vi "LJUD UE9RAW SingleIO.vi"(5 "Comm Settings":T1={"Open LabJack "=TRUE, "Use USB"=TRUE, "IP Address"="192.168.1.209", "PortA"=52360, "PortB"=0}, 8 "error in (no error)":errorcluster, 10 "Write Parameters":T3 {"IOType" items=["Digital Bit In", "Digital Bit Out", "Digital Port In", "Digital Port Out", "Analog In", "Analog Out"]}, 11 "Handle In":i32) -> (0 "error out":errorcluster, 2 "Read Parameters":T2 {"IOType" items=["Digital Bit In", "Digital Bit Out", "Digital Port In", "Digital Port Out", "Analog In", "Analog Out"]}, 3 "Handle Out":i32)   [LabVIEW 2021]
panel:
  # "Digital Port\nChannel:\n0  =  FIO\n1  =  EIO\n2  =  CIO\n3  =  MIO"
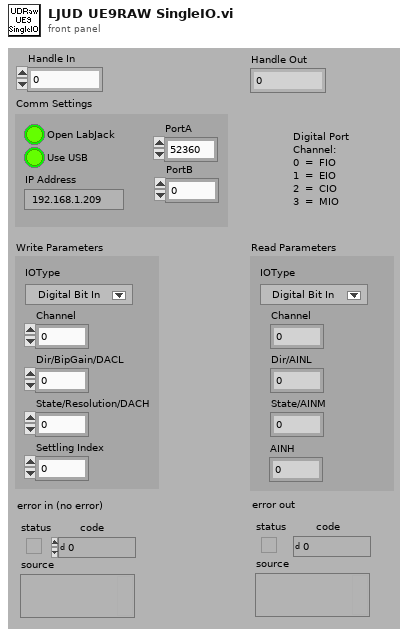
[diagram p1: front panel]
types:
  T1 = cluster{"Open LabJack ":bool, "Use USB":bool, "IP Address":string, "PortA":u16, "PortB":u16}
  T2 = cluster{"IOType":u16, "Channel":u8, "Dir/AINL":u8, "State/AINM":u8, "AINH":u8}
  T3 = cluster{"IOType":u8, "Channel":u8, "Dir/BipGain/DACL":u8, "State/Resolution/DACH":u8, "Settling Index":u8}
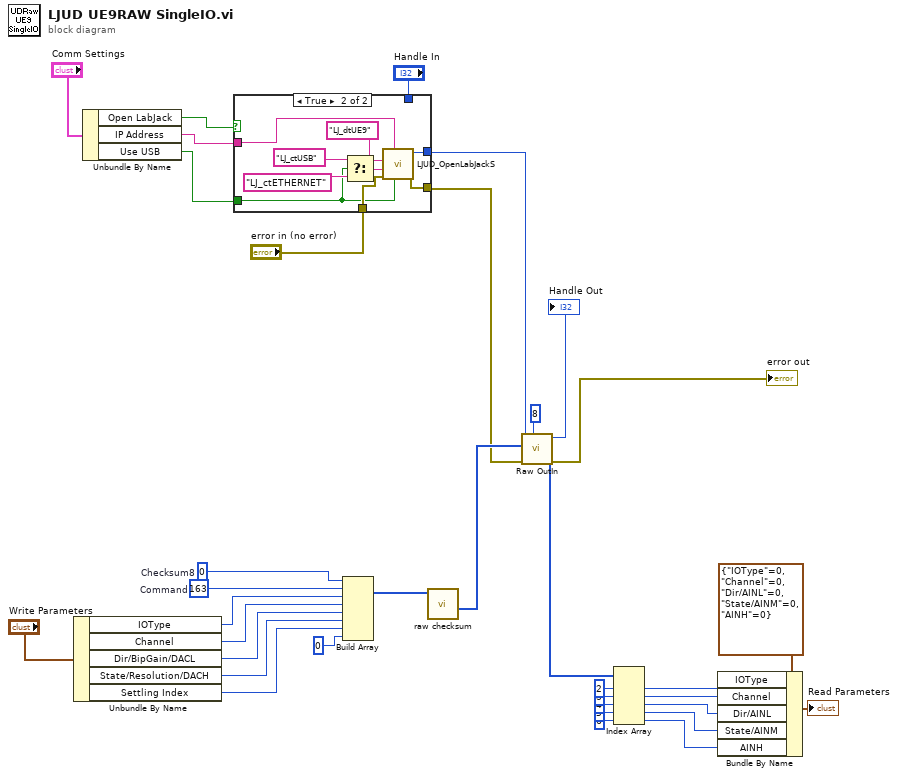
[diagram p0: block diagram]
diagram:
  w33 = u8 0  # Checksum8
  w35 = u8 163  # Command
  n1 = Unbundle By Name("Write Parameters") -> ("IOType"=w30:u8, "Channel"=w29:u8, "Dir/BipGain/DACL"=w28:u8, "State/Resolution/DACH"=w27:u8, "Settling Index"=w26:u8)
  n2 = Unbundle By Name("Comm Settings") -> ("Open LabJack"=w7:bool, "IP Address"=w6:string, "Use USB"=w5:bool)
  n3 = case shown="True" w7 {
    tunnel: w6 -> [_ w40]
    tunnel: "error in (no error)" -> [w37 w44]
    tunnel: [w37 w43] -> w3
    tunnel: [w36 w41] -> w2
    tunnel: w5 -> [_ w42]
    tunnel: "Handle In" -> [w36 _]
    frame False {
    }
    frame True {
      n4 = Select(t="LJ_ctUSB" ("ConnectionType"), s=w42, f="LJ_ctETHERNET" ("ConnectionType")) -> (s? t:f=w38:string)
      n5 = call "LJUD_OpenLabJackS.vi"("FirstFound"=w42, "Address"=w40, "error in"=w44, "ConnectionType"=w38, "DeviceType"="LJ_dtUE9") -> ("error out"=w43:errorcluster, "Handle"=w41:i32)  [unwired: 4 in, 1 out]
    }
  }
  n6 = Build Array(w33, w35, w30, w29, w28, w27, w26, u8 0 ("Input Element")) -> (w34:u8[])
  n7 = call "raw checksum.vi"("Array"=w34) -> ("Array Output"=w32:u8[])  [unwired: 3 in, 7 out]
  n8 = call "Raw OutIn.vi"("# of bytes to read in"=8 ("# of bytes to read"), "error in"=w3, "Raw Out"=w32, "Handle In"=w2) -> ("error out"=→"error out":errorcluster, "Raw In"=w24:u8[], "Handle Out"=→"Handle Out":i32)  [unwired: 4 in, 1 out]
  n9 = Index Array(array=w24, index #1=2 ("Index"), index #2=3 ("Index"), index #3=4 ("Index"), index #4=5 ("Index"), index #5=6 ("Index")) -> (element #1=w23:u8, element #2=w22:u8, element #3=w21:u8, element #4=w14:u8, element #5=w12:u8)
  n10 = Bundle By Name(cluster=T2 {"IOType"=0, "Channel"=0, "Dir/AINL"=0, "State/AINM"=0, "AINH"=0} ("Read Parameters"), "IOType"=w23, "Channel"=w22, "Dir/AINL"=w21, "State/AINM"=w14, "AINH"=w12) -> (→"Read Parameters":T2)
